vi "Initialize.vi"(8 "error in":errorcluster, 10 "DataType":refnum<class "Data.lvclass">, 11 "Data Subject in":refnum<class "Publisher.lvclass">) -> (0 "error out":errorcluster, 2 "DVR":refnum<data-value>, 3 "Data Subject out":refnum<class "Publisher.lvclass">)   [LabVIEW 2014, in "Publisher.lvclass"]
doc: "This VI must be overridden to provide useful feedback but the parent will provide a reference for a stop occurrence that can be used by the children. Children should provide a reference to the proper data object (loading it into the subject class). The specific data object must be downcasted to the generic data object."
uses:
  Publisher.lvclass
  Data/Data.lvclass
  Publisher.lvclass/Publisher.ctl
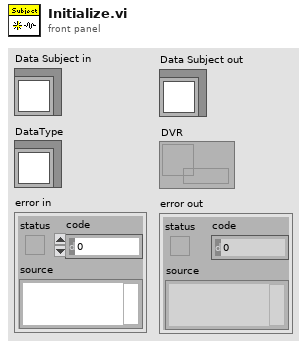
[diagram p1: front panel]
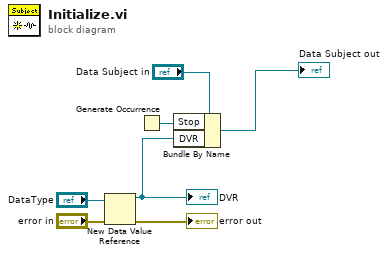
[diagram p0: block diagram]
diagram:
  n1 = New Data Value Reference(data value="DataType", error in="error in") -> (data value reference=w1:refnum<data-value>, error out=→"error out":errorcluster)
  "DVR" <- w1
  n2 = Generate Occurrence() -> (w5:refnum<k4>)
  n3 = Bundle By Name(cluster="Data Subject in", "Stop"=w5, "DVR"=w1) -> (→"Data Subject out":refnum<class "Publisher.lvclass">)
